vi "Register for gRPC Server Events.vi"(8 "error in (no error)":errorcluster, 11 "CIFCorePlugin in":refnum<class "CIFCorePlugin.lvclass">) -> (0 "error out":errorcluster, 2 "Event Registration Refnum":refnum<event-registration>, 3 "CIFCorePlugin out":refnum<class "CIFCorePlugin.lvclass">)   [LabVIEW 2021, in "CIFCorePlugin.lvclass"]
uses:
  CIFCorePlugin.lvclass
  Grpc/CIFCorePlugin_server/RPC Service/PluginCore/PluginCore.lvclass
  Grpc/CIFCoreChannel_server/RPC Service/ChannelCore/ChannelCore.lvclass
  C:/Program Files/National Instruments/LabVIEW 2021/vi.lib/gRPC/LabVIEW gRPC Servicer/ServiceBase/ServiceBase.lvclass
  <vilib>/gRPC/LabVIEW gRPC Library/Shared/grpcId.ctl
  <vilib>/gRPC/LabVIEW gRPC Library/grpc-lvsupport-release.lvlib
  <vilib>/gRPC/LabVIEW gRPC Library/Server API/typeDefs/gRPCId Cluster.ctl
  Grpc/CIFCorePlugin_server/RPC Service/PluginCore/typeDefs/Server gRPC UEs.ctl
  Grpc/CIFCoreChannel_server/RPC Service/ChannelCore/typeDefs/Server gRPC UEs.ctl
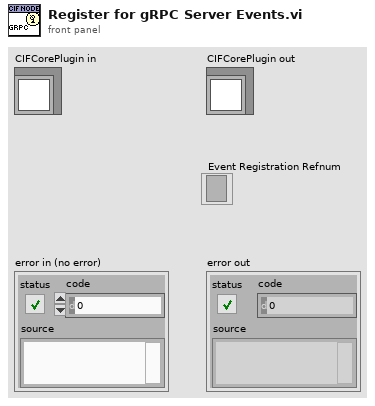
[diagram p1: front panel]
types:
  T1 = typedef "CIFCorePlugin_server.lvlib/PluginCore.lvclass/Server gRPC UEs.ctl" = cluster{"PluginCore Start gRPC UE":refnum<user-event>, "PluginCore Pause gRPC UE":refnum<user-event>, "PluginCore Stop gRPC UE":refnum<user-event>, "PluginCore RefreshStatistics gRPC UE":refnum<user-event>, "PluginCore UpdateConfig gRPC UE":refnum<user-event>, "PluginCore GetStatusData gRPC UE":refnum<user-event>, "PluginCore GetVersion gRPC UE":refnum<user-event>, "PluginCore GetConfig gRPC UE":refnum<user-event>, "PluginCore GetOverrides gRPC UE":refnum<user-event>}
  T2 = typedef "CIFCoreChannel_server.lvlib/ChannelCore.lvclass/Server gRPC UEs.ctl" = cluster{"ChannelCore GetChannels gRPC UE":refnum<user-event>, "ChannelCore SetConnection gRPC UE":refnum<user-event>, "ChannelCore SetForce gRPC UE":refnum<user-event>}
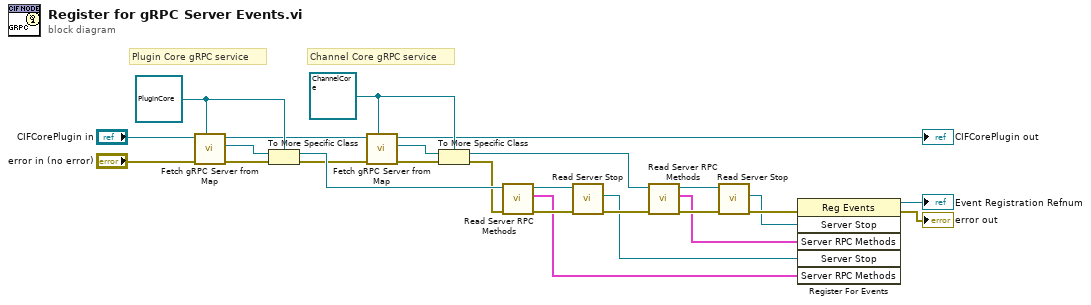
[diagram p0: block diagram]
diagram:
  w12 = refnum<class "ChannelCore.lvclass"> refnum ("CIFCoreChannel_server.lvlib:ChannelCore.lvclass")
  w22 = refnum<class "PluginCore.lvclass"> refnum ("CIFCorePlugin_server.lvlib:PluginCore.lvclass")
  # "Channel Core gRPC service"
  # "Plugin Core gRPC service"
  n1 = call "Fetch gRPC Server from Map.vi"("gRPC Server Class type"=w22, "error in (no error)"="error in (no error)", "CIFCorePlugin in"="CIFCorePlugin in") -> ("error out"=w21:errorcluster, "gRPC Server Class out"=w20:refnum<class "ServiceBase.lvclass">, "CIFCorePlugin out"=w15:refnum<class "CIFCorePlugin.lvclass">)  [unwired: 6 in]
  n2 = To More Specific Class(target class=w22, reference=w20, error in=w21) -> (specific class reference=w23:refnum<class "PluginCore.lvclass">, error out=w14:errorcluster)
  n3 = call "Fetch gRPC Server from Map.vi"("gRPC Server Class type"=w12, "error in (no error)"=w14, "CIFCorePlugin in"=w15) -> ("error out"=w16:errorcluster, "gRPC Server Class out"=w17:refnum<class "ServiceBase.lvclass">, "CIFCorePlugin out"=→"CIFCorePlugin out":refnum<class "CIFCorePlugin.lvclass">)  [unwired: 6 in]
  n4 = To More Specific Class(target class=w12, reference=w17, error in=w16) -> (specific class reference=w9:refnum<class "ChannelCore.lvclass">, error out=w3:errorcluster)
  n5 = call "Read Server RPC Methods.vi"("error in (no error)"=w3, "SignalGeneratorService in"=w23) -> ("error out"=w24:errorcluster, "Server RPC Methods"=w7:T1, "SignalGeneratorService out"=w25:refnum<class "PluginCore.lvclass">)  [unwired: 7 in]
  n6 = call-dynamic "Read Server Stop.vi"("error in"=w24, "iService in"=w25) -> ("error out"=w11:errorcluster, "Server Stop"=w6:refnum<user-event>)  [unwired: 7 in, 1 out]
  n7 = call "Read Server RPC Methods.vi"("error in (no error)"=w11, "SignalGeneratorService in"=w9) -> ("error out"=w13:errorcluster, "Server RPC Methods"=w5:T2, "SignalGeneratorService out"=w8:refnum<class "ChannelCore.lvclass">)  [unwired: 7 in]
  n8 = call-dynamic "Read Server Stop.vi"("error in"=w13, "iService in"=w8) -> ("error out"=w10:errorcluster, "Server Stop"=w4:refnum<user-event>)  [unwired: 7 in, 1 out]
  n9 = register-events(error in=w10, w4, w5, w6, w7) -> (reference out=→"Event Registration Refnum":refnum<event-registration>, error out=→"error out":errorcluster)  [unwired: 1 in]
